vi "DAQmx Write (Digital 1D U8 1Chan NSamp).vi"(0 "task/channels in":refnum<k21>, 1 "auto start":bool, 7 "data":u8[](array[numeric]), 9 "timeout":dbl=10.0 format="%0.2f", 11 "error in":errorcluster) -> (4 "task out":refnum<k21>, 10 "number of samples written per channel":u32, 15 "error out":errorcluster)   [LabVIEW 2017]
doc: "Writes one or more 8-bit unsigned integer samples to a task that contains a single digital output channel. Use an instance that writes 8-bit unsigned integers for devices with up to eight lines per port."
uses:
  nilvaiu.dll
panel:
  # "sample #"
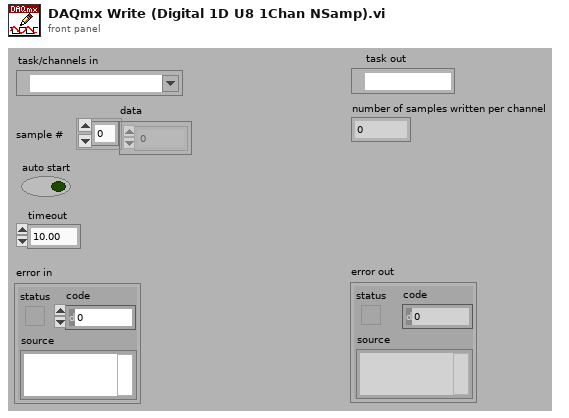
[diagram p1: front panel]
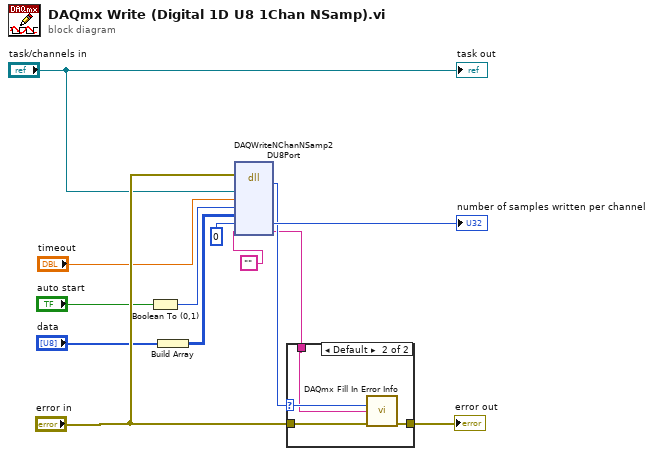
[diagram p0: block diagram]
diagram:
  n1 = Boolean To (0,1)(Boolean="auto start") -> (0, 1=w5:i16)
  n2 = Build Array("data") -> (w1:u8[][])
  n3 = dll-call lib="nilvaiu.*" fn="DAQWriteNChanNSamp2DU8Port"(error in="error in", "taskID"="task/channels in", "timeout"="timeout", "autoStart"=w5, "data"=w1, "numSamplesWriten"=u32 0, "extendedErrorInfo"="") -> (w6:i32, "numSamplesWriten"=→"number of samples written per channel":u32, "extendedErrorInfo"=w4:string)  [unwired: 4 in, 4 out]
  n4 = case shown="Default" w6 {
    selector: w6 -> [_ w16]
    tunnel: "error in" -> [w14 w18]
    tunnel: [w14 w17] -> w11
    tunnel: w4 -> [_ w15]
    frame 0 {
    }
    frame Default {
      n5 = call "DAQmx Fill In Error Info.vi"("status code"=w16, "extended error info"=w15, "error in"=w18) -> ("error out"=w17:errorcluster)  [unwired: 1 in, 11 out]
    }
  }
  "error out" <- w11
  "task out" <- "task/channels in"
